vi "Example.vi"() -> ()   [LabVIEW 2015]
uses:
  Stop.vi
  Gates/Gates.lvlib
panel:
  out "gate name":string
  out "# waiting for open gate":i32
  out "process 6":bool
  out "process 5":bool
  out "process 4":bool
  out "process 3":bool
  out "process 2":bool
  out "process 1":bool
  in  "stop":bool
  in  "open":bool
  in  "close":bool
  # "See block diagram for description."
  # "Interface"
  # "Display"
  # "Status"
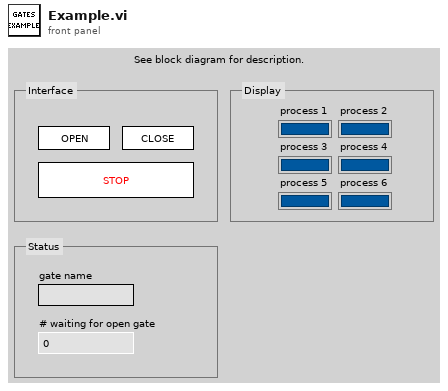
[diagram p1: front panel]
types:
  T1 = typedef "Gates.lvlib/Gate.ctl" = refnum<k1>
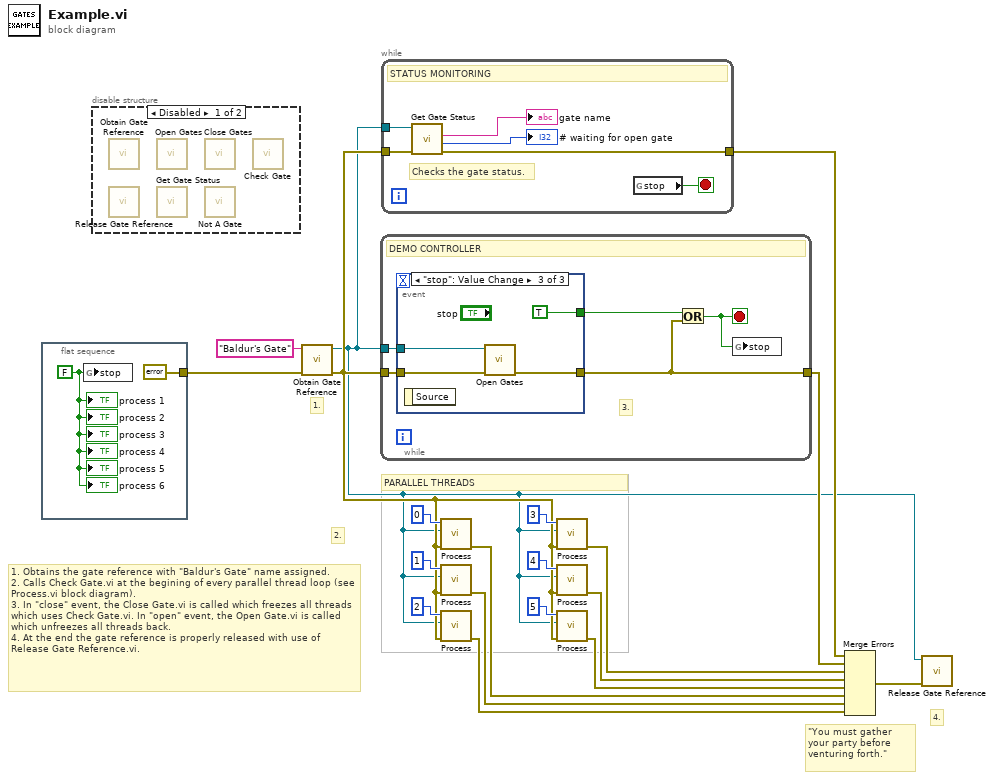
[diagram p0: block diagram]
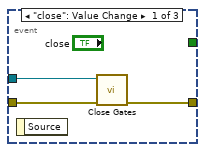
[diagram p3: hidden frame]
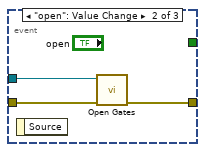
[diagram p4: hidden frame]
diagram:
  # "\"You must gather your party before venturing forth.\""
  # "1. Obtains the gate reference with \"Baldur's Gate\" name assigned.\n2. Calls Check Gate.vi at the begining of every parallel thread loop (see Process.vi block diagram).\n3. In \"close\" event, the Close Gate.vi is called which freezes all threads which uses Check Gate.vi. In \"open\" event, the Open Gate.vi is called which unfreezes all threads back.\n4. At the end the gate reference is properly released with use of Release Gate Reference.vi."
  # "4."
  # "2."
  # "1."
  # "PARALLEL THREADS"
  n1 = flat-sequence {
    tunnel: [errorcluster {"status"=FALSE, "code"=0, "source"=""} ("error in (no error)")] -> w7
    frame #0 {
      w20 = FALSE ("stop")
      n2 = global write "Stop.vi" "stop"(w20) -> ()
      "process 1" <- w20
      "process 2" <- w20
      "process 6" <- w20
      "process 4" <- w20
      "process 3" <- w20
      "process 5" <- w20
    }
  }
  n3 = disable-structure shown="Disabled" {
    frame Disabled {
      n4 = call "Obtain Gate Reference.vi"() -> ()  [unwired: 8 in, 3 out]
      n5 = call "Release Gate Reference.vi"() -> ()  [unwired: 10 in, 2 out]
      n6 = call "Open Gates.vi"() -> ()  [unwired: 10 in, 2 out]
      n7 = call "Get Gate Status.vi"() -> ()  [unwired: 8 in, 4 out]
      n8 = call "Close Gates.vi"() -> ()  [unwired: 10 in, 2 out]
      n9 = call "Not A Gate.vi"() -> ()  [unwired: 1 in, 1 out]
      n10 = call "Check Gate.vi"() -> ()  [unwired: 9 in, 3 out]
    }
    frame Enabled {
    }
  }
  n11 = call "Obtain Gate Reference.vi"("name (unnamed)"="Baldur's Gate", "error in (no error)"=w7) -> ("gate"=w1:T1, "error out"=w4:errorcluster)  [unwired: 6 in, 1 out]
  n12 = while {
    tunnel: w4 -> [w26]
    tunnel: [w23] -> w5
    tunnel: w1 -> [w25]
    stop <- w22 stop-if-true
    # "3."
    # "DEMO CONTROLLER"
    n13 = event shown="[2] \"stop\": Value Change" {
      selector: _ -> [_ _ _]
      dyn-events: _ -> [_ _ _]
      timeout: _ -> [_ _ _]
      tunnel: [_ _ TRUE] -> w24
      tunnel: w26 -> [w29 w32 w35]
      tunnel: [w27 w30 w33] -> w23
      tunnel: w25 -> [w28 w31 w34]
      event "close": Value Change {
        n14 = event-data() -> ()  [unwired: 1 in, 1 out]
        n15 = call "Close Gates.vi"("error in (no error)"=w29, "gate"=w28) -> ("error out"=w27:errorcluster)  [unwired: 8 in, 1 out]
      }
      event "open": Value Change {
        n16 = event-data() -> ()  [unwired: 1 in, 1 out]
        n17 = call "Open Gates.vi"("error in (no error)"=w32, "gate"=w31) -> ("error out"=w30:errorcluster)  [unwired: 8 in, 1 out]
      }
      event "stop": Value Change {
        n18 = event-data() -> ()  [unwired: 1 in, 1 out]
        n19 = call "Open Gates.vi"("error in (no error)"=w35, "gate"=w34) -> ("error out"=w33:errorcluster)  [unwired: 8 in, 1 out]
      }
    }
    n20 = Or(x=w24, y=w23) -> (x .or. y?=w22:bool)
    n21 = global write "Stop.vi" "stop"(w22) -> ()
  }
  n22 = while {
    tunnel: w1 -> [w42]
    tunnel: w4 -> [w41]
    tunnel: [w40] -> w3
    stop <- w37 stop-if-true
    # "Checks the gate status."
    # "STATUS MONITORING"
    n23 = call "Get Gate Status.vi"("error in (no error)"=w41, "gate"=w42) -> ("error out"=w40:errorcluster, "# waiting for open gate"=→"# waiting for open gate":i32, "gate name"=→"gate name":string)  [unwired: 6 in, 1 out]
    n24 = global read "Stop.vi" "stop"() -> (w37:bool)
  }
  n25 = call "Process.vi"("error in (no error)"=w4, "gate"=w1, "process index"=0) -> ("error out"=w11:errorcluster)  [unwired: 8 in]
  n26 = call "Process.vi"("error in (no error)"=w4, "gate"=w1, "process index"=1) -> ("error out"=w12:errorcluster)  [unwired: 8 in]
  n27 = call "Process.vi"("error in (no error)"=w4, "gate"=w1, "process index"=2) -> ("error out"=w13:errorcluster)  [unwired: 8 in]
  n28 = call "Process.vi"("error in (no error)"=w4, "gate"=w1, "process index"=3) -> ("error out"=w8:errorcluster)  [unwired: 8 in]
  n29 = call "Process.vi"("error in (no error)"=w4, "gate"=w1, "process index"=4) -> ("error out"=w9:errorcluster)  [unwired: 8 in]
  n30 = call "Process.vi"("error in (no error)"=w4, "gate"=w1, "process index"=5) -> ("error out"=w10:errorcluster)  [unwired: 8 in]
  n31 = Merge Errors(w3, w5, w8, w9, w10, w11, w12, w13) -> (w6:errorcluster)
  n32 = call "Release Gate Reference.vi"("error in (no error)"=w6, "gate"=w1) -> ()  [unwired: 8 in, 2 out]
